vi "UpdateActualDepsOfLibraries.vi"(4 "Overall Status Indicator Ref":refnum<vi>, 6 "Status Indicator Ref":refnum<vi>, 8 "error in (no error)":errorcluster, 9 "Repo/Workspace Path":path, 10 "Lvlib / Class Names":string[](array[string]), 11 "CLI in":refnum<class "CLI.lvclass">) -> (0 "error out":errorcluster, 3 "CLI out":refnum<class "CLI.lvclass">)   [LabVIEW 2019, in "Hawkeye.lvlib"]
uses:
  Hawkeye.lvlib
  <vilib>/Wiresmith Technology/G CLI/CLI Class/CLI.lvclass
  <vilib>/Utility/config.llb/NI_LVConfig.lvlib
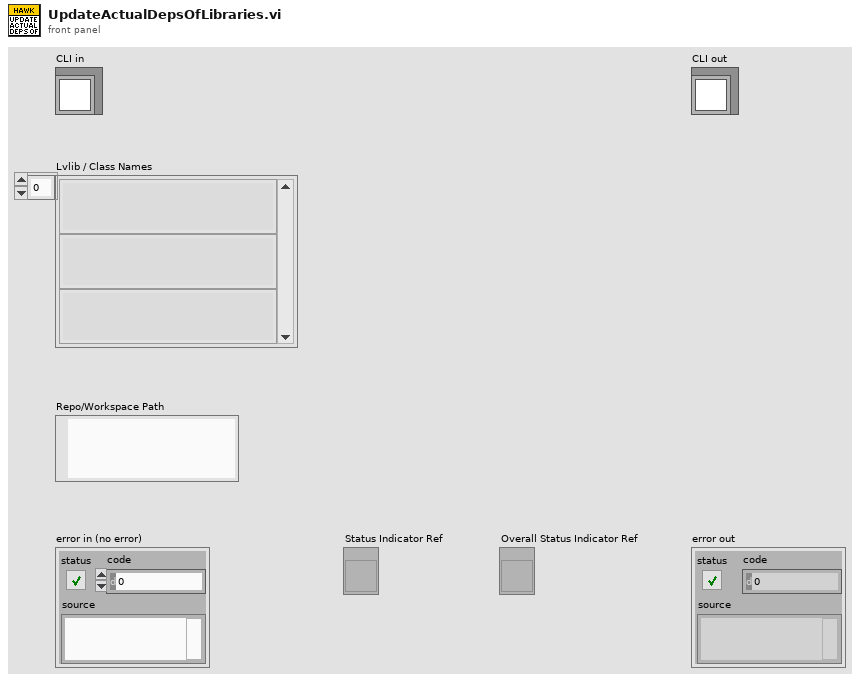
[diagram p1: front panel]
types:
  T1 = typedef "NI_LVConfig.lvlib/Config Data RefNum.ctl" = refnum<k1>
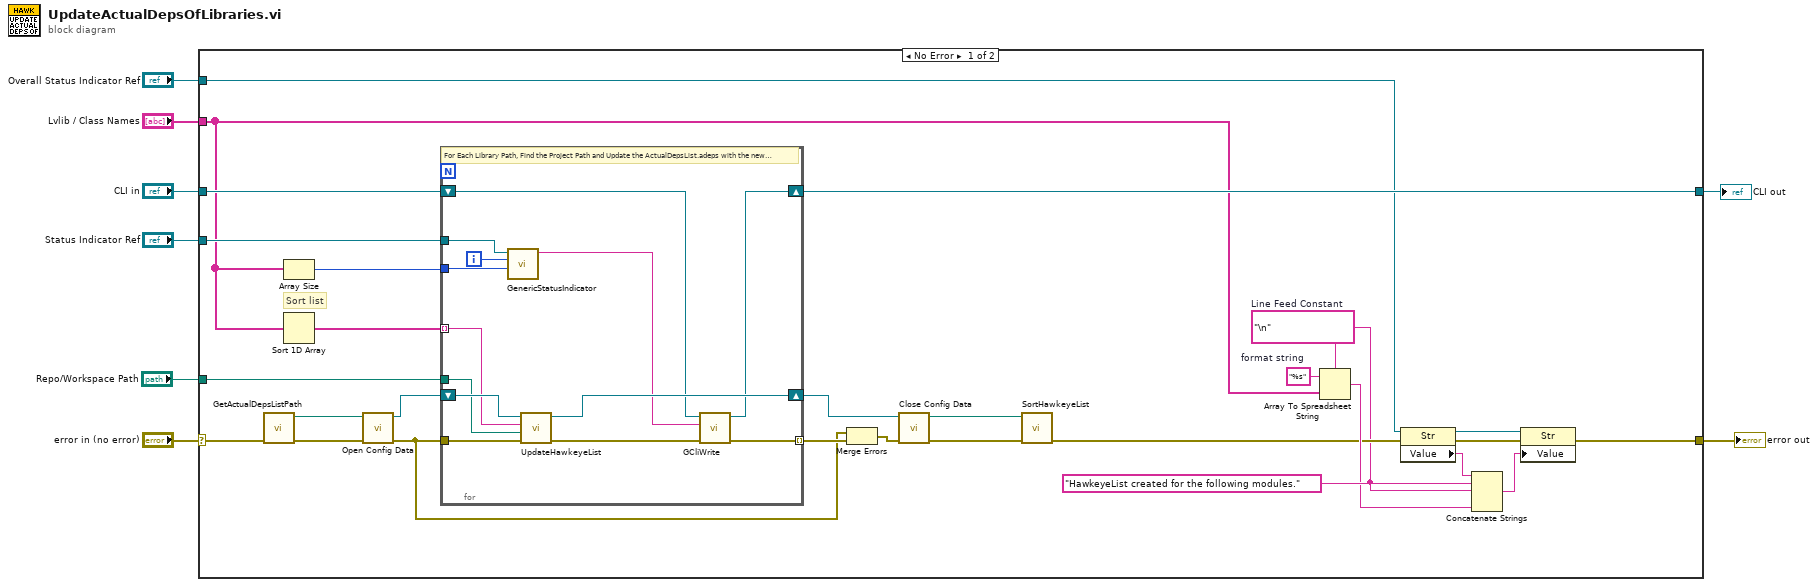
[diagram p0: block diagram]
diagram:
  n1 = case shown="No Error" "error in (no error)" {
    selector: "error in (no error)" -> [w27 w51]
    tunnel: "Status Indicator Ref" -> [w22 _]
    tunnel: [w20 w51] -> w7
    tunnel: [w36 w50] -> w6
    tunnel: "CLI in" -> [w35 w50]
    tunnel: "Lvlib / Class Names" -> [w16 _]
    tunnel: "Overall Status Indicator Ref" -> [w11 _]
    tunnel: "Repo/Workspace Path" -> [w15 _]
    frame No Error {
      w9 = "\n"  # Line Feed Constant
      w18 = "%s"  # format string
      # "Sort list"
      n2 = call "GetActualDepsListPath.vi"("error in (no error)"=w27) -> ("error out"=w34:errorcluster, "ActualDepsListPath"=w33:path)  [unwired: 9 in]
      n3 = Array Size(array=w16) -> (size(s)=w31:i32)
      n4 = Sort 1D Array(array=w16) -> (sorted array=w25:string[])
      n5 = call <vilib>:"Open Config Data.vi"("error in (no error)"=w34, "configuration file path"=w33) -> ("error out"=w26:errorcluster, "refnum"=w32:T1)  [unwired: 7 in, 1 out]
      n6 = for {
        tunnel: w26 -> [w49]
        tunnel: [w43] -> w28 mode=indexing
        shift-right: [w47] -> w30
        shift-left: w32 -> [w48]
        tunnel: w31 -> [w46]
        shift-right: [w42] -> w36
        shift-left: w35 -> [w41]
        tunnel: w22 -> [w38]
        tunnel: w25 -> [w39] mode=indexing
        tunnel: w15 -> [w37]
        i -> [w45]
        # "For Each Library Path, Find the Project Path and Update the ActualDepsList.adeps with the new dependencies found"
        n7 = call "GenericStatusIndicator.vi"("Total"=w46, "Current Iteration"=w45, "Status Indicator Ref In"=w38) -> ("CLI Status to Print"=w40:string)  [unwired: 8 in]
        n8 = call "UpdateHawkeyeList.vi"("error in (no error)"=w49, "Repo/Workspace Path"=w37, "Library/Class Name"=w39, "Config Refnum in"=w48) -> ("error out"=w44:errorcluster, "Config Refnum out"=w47:T1)  [unwired: 4 in, 2 out]
        n9 = call "GCliWrite.vi"("error in (no error)"=w44, "Text to Write"=w40, "CLI in"=w41) -> ("error out"=w43:errorcluster, "CLI out"=w42:refnum<class "CLI.lvclass">)  [unwired: 7 in]
      }
      n10 = Merge Errors(w26, w28) -> (w29:errorcluster)
      n11 = call <vilib>:"Close Config Data.vi"("error in (no error)"=w29, "refnum"=w30) -> ("error out"=w23:errorcluster, "file path"=w24:path)  [unwired: 8 in]
      n12 = call "SortHawkeyeList.vi"("error in (no error)"=w23, "Hawkeye File Path"=w24) -> ("error out"=w14:errorcluster)  [unwired: 8 in, 1 out]
      n13 = Array To Spreadsheet String(delimiter (Tab)=w9, array=w16, 3:w18) -> (spreadsheet string=w17:string)
      n14 = property class="Str"(reference=w11, error in=w14) -> (reference out=w12:refnum<vi>, error out=w13:errorcluster, "Value"=w10:string)
      n15 = Concatenate Strings(w10, "HawkeyeList created for the following modules." ("string"), w9, w9, w17) -> (w19:string)
      n16 = property class="Str"(reference=w12, error in=w13, "Value"=w19) -> (error out=w20:errorcluster)  [unwired: 1 out]
    }
    frame Error {
    }
  }
  "error out" <- w7
  "CLI out" <- w6
